vi "TempMonitor_SetTempInput_ConfirmDUTtempSerial.vi"(8 "Temp Tolerance (C)":dbl=1.5 min=0.0 max=5.0 step=0.01 format="%0.2f", 9 "Sensor Temp (C)":dbl=10.0 min=-25.0 max=100.0 step=1.0 format="%0.2f", 10 "Test Block Analog Output":tag="Dev1/ao0", 11 "Serial Port to Use":refnum<visa-resource-name>="COM8") -> (0 "Error Out":errorcluster, 1 "Response":string, 2 "Device Temp (C)":dbl=-1000.0, 3 "Pass":bool)   [LabVIEW 2012]
doc: "Set an analog voltage as input to the DUT using the USB-6008 device. Then over UART read from the DUT what temperature it read."
uses:
  <vilib>/DAQmx/write.llb/DAQmx Write (Analog DBL 1Chan 1Samp).vi
  TempMonitor_Command_Enumerations.vi
  <vilib>/DAQmx/create/channels.llb/DAQmx Create Channel (AO-Voltage-Basic).vi
  <vilib>/DAQmx/miscellaneous.llb/DAQmx Fill In Error Info.vi
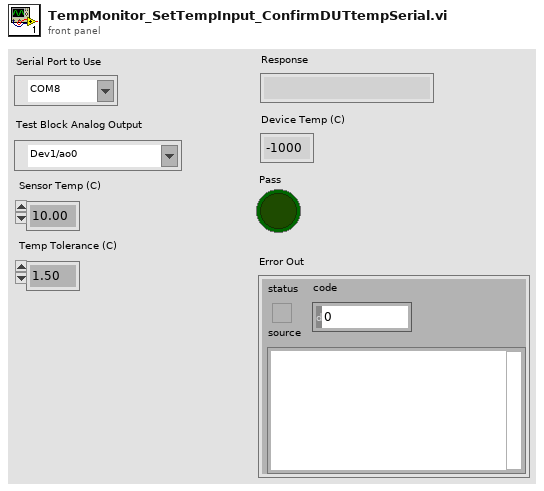
[diagram p1: front panel]
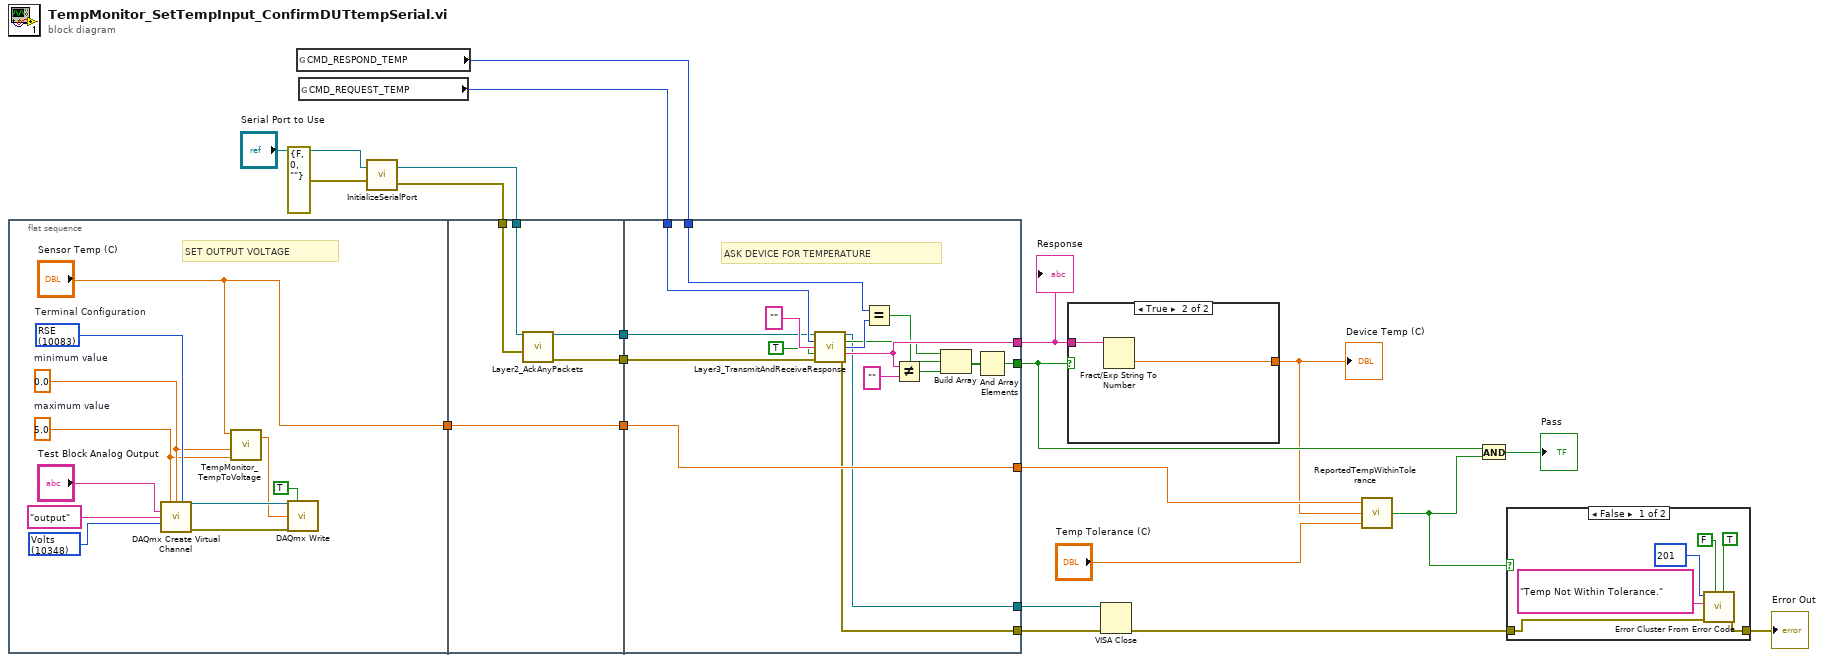
[diagram p0: block diagram]
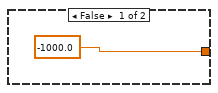
[diagram p3: hidden frame]
diagram:
  n1 = flat-sequence {
    tunnel: ["Sensor Temp (C)"] -> w15
    tunnel: [w37] -> w16
    tunnel: w13 -> [w36]
    tunnel: w15 -> [w37]
    tunnel: w11 -> [w35]
    tunnel: [w34] -> w10
    tunnel: [w33] -> w9
    tunnel: [w49] -> w21
    tunnel: [w54] -> w20
    tunnel: w16 -> [w42]
    tunnel: [w42] -> w6
    tunnel: w18 -> [w48]
    tunnel: w17 -> [w46]
    tunnel: w10 -> [w41]
    tunnel: w9 -> [w40]
    tunnel: [w39] -> w8
    tunnel: [w38] -> w7
    frame #0 {
      w26 = 10083 items=["Default"=-1, "RSE"=10083, "Differential"=10106, "Pseudodifferential"=12529]  # Terminal Configuration
      w23 = 5.0  # maximum value
      w24 = 0.0  # minimum value
      w27 = 10348 items=["Volts"=10348, "From Custom Scale"=10065] ("units")
      # "SET OUTPUT VOLTAGE"
      n2 = call-poly <vilib>:"DAQmx Create Virtual Channel.vi"("maximum value"=w23, "minimum value"=w24, "output terminal configuration"=w26, "physical channels"="Test Block Analog Output", "name to assign"="output", "units"=w27) -> ("task out"=w32:refnum<k21>, "error out"=w31:errorcluster)  [unwired: 8 in]
      n3 = call "TempMonitor_TempToVoltage.vi"("Max Voltage"=w23, "Min Voltage"=w24, "Temp (C)"="Sensor Temp (C)") -> ("Output Voltage"=w22:dbl)  [unwired: 1 in, 1 out]
      n4 = call-poly <vilib>:"DAQmx Write.vi"("task/channels in"=w32, "auto start"=TRUE, "data"=w22, "error in"=w31) -> ()  [unwired: 9 in, 3 out]
    }
    frame #1 {
      n5 = call "Layer2_AckAnyPackets.vi"("Serial Port to Use"=w36, "Error In"=w35) -> ("Serial Port to Use (out)"=w34:refnum<visa-resource-name>, "Error Out"=w33:errorcluster)  [unwired: 9 in, 3 out]
    }
    frame #2 {
      # "ASK DEVICE FOR TEMPERATURE"
      n6 = call "Layer3_TransmitAndReceiveResponse.vi"("Serial Port to Use"=w41, "CMD"=w48, "Message"="", "Expecting Response"=TRUE, "error in (no error)"=w40) -> ("Serial Port to Use (out)"=w38:refnum<visa-resource-name>, "Success"=w44:bool, "Response CMD"=w45:u16, "Response Message"=w49:string, "Error Out"=w39:errorcluster)  [unwired: 6 in]
      n7 = Equal?(x=w46, y=w45) -> (x = y?=w43:bool)
      n8 = Not Equal?(x=w49, y="" ("x")) -> (x != y?=w47:bool)
      n9 = Build Array(w44, w43, w47) -> (w53:bool[])
      n10 = And Array Elements(Boolean array=w53) -> (logical AND=w54:bool)
    }
  }
  n11 = global read "TempMonitor_Command_Enumerations.vi" "CMD_RESPOND_TEMP"() -> (w17:u16)
  n12 = global read "TempMonitor_Command_Enumerations.vi" "CMD_REQUEST_TEMP"() -> (w18:u16)
  n13 = call "InitializeSerialPort.vi"("error in (no error)"=errorcluster {"status"=FALSE, "code"=0, "source"=""} ("Error In"), "Serial Port to Use"="Serial Port to Use") -> ("error out"=w11:errorcluster, "Configured Serial Port Identifier"=w13:refnum<visa-resource-name>)
  n14 = case shown="True" w20 {
    tunnel: w21 -> [_ w57]
    tunnel: [-1000.0 w56] -> w5
    frame False {
    }
    frame True {
      n15 = Fract/Exp String To Number(string=w57) -> (number=w56:dbl)  [unwired: 3 in, 1 out]
    }
  }
  "Device Temp (C)" <- w5
  n16 = VISA Close(VISA resource name=w7, error in (no error)=w8) -> (error out=w2:errorcluster)
  n17 = call "ReportedTempWithinTolerance.vi"("Temp Tolerance (C)"="Temp Tolerance (C)", "Set Temp (C)"=w5, "Reported Temp (C)"=w6) -> ("Pass"=w3:bool)
  n18 = And(x=w20, y=w3) -> (x .and. y?=→"Pass":bool)
  n19 = case shown="False" w3 {
    tunnel: w2 -> [w58 w64]
    tunnel: [w61 w64] -> w1
    frame False {
      n20 = call <vilib>:"Error Cluster From Error Code.vi"("is warning? (False)"=TRUE, "show call chain? (False)"=FALSE, "error in (no error)"=w58, "error message (\"\")"="Temp Not Within Tolerance." ("source"), "error code (0)"=201 ("code")) -> ("error out"=w61:errorcluster)  [unwired: 4 in]
    }
    frame True {
    }
  }
  "Error Out" <- w1
  "Response" <- w21
